vi "MakeTDtargVI.vi"() -> ()   [LabVIEW 2024]
panel:
  in  "String":string
  in  "asdf":dbl
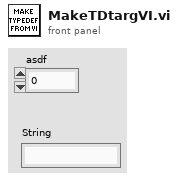
[diagram p1: front panel]
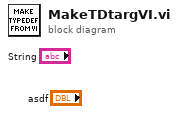
[diagram p0: block diagram]
diagram:
